vi "S2C_PCIe7841_Proc_DigitalWriteLocal.vi"(8 "Error In":errorcluster, 9 "ExeRef":refnum<vi>, 11 "Q-Ref":refnum<queue>) -> (0 "Error Out":errorcluster, 3 "Command":string)   [LabVIEW 2015]
uses:
  Typedefs/S2C_PCIe7841_Type_Conn0Write.ctl
  Typedefs/S2C_PCIe7841_Type_Conn1Write.ctl
  Typedefs/S2C_PCIe7841_Type_Conn2Write.ctl
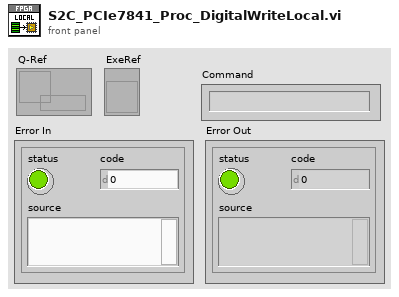
[diagram p1: front panel]
types:
  T1 = cluster{"Caller-Q":refnum<queue>, "Command":string, "Return":string, "Data":variant, "Timeout":dbl}
  T2 = typedef "S2C_PCIe7841_Type_Conn0Write.ctl" = u16
  T3 = typedef "S2C_PCIe7841_Type_Conn1Write.ctl" = u16
  T4 = typedef "S2C_PCIe7841_Type_Conn2Write.ctl" = u16
  T5 = cluster{"Connector":u16, "Conn0_Item":T2, "Conn1_Item":T3, "Conn2_Item":T4, "State":bool, "P5C1Exe":bool}
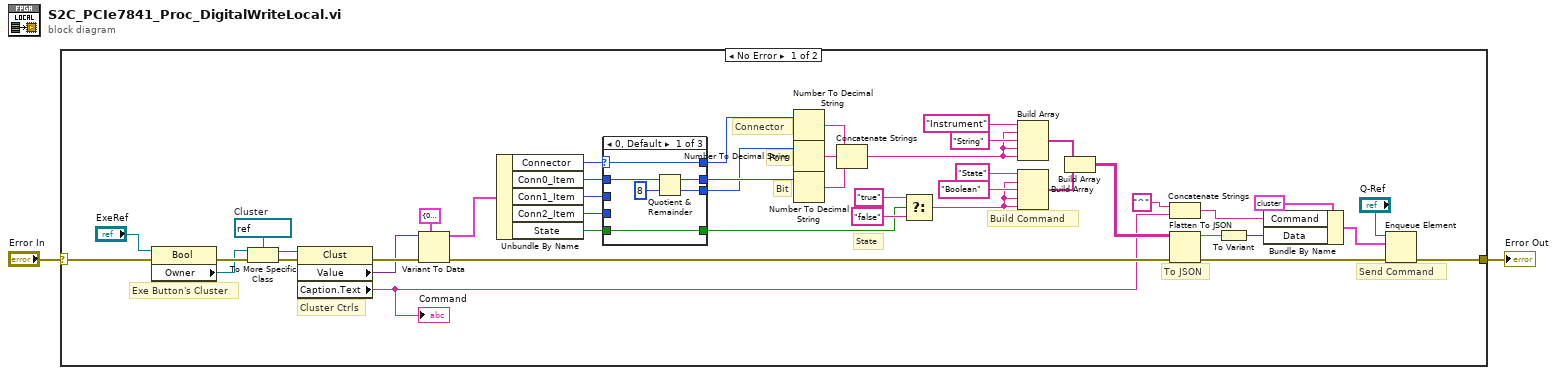
[diagram p0: block diagram]
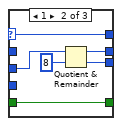
[diagram p2: hidden frame]
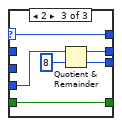
[diagram p3: hidden frame]
diagram:
  n1 = case shown="No Error" "Error In" {
    selector: "Error In" -> [w41 w66]
    tunnel: [w40 w66] -> w1
    frame No Error {
      w44 = refnum<vi> refnum  # Cluster
      # "Build Command"
      # "State"
      # "Bit"
      # "Port"
      # "Connector"
      # "Send Command"
      # "To JSON"
      # "Cluster Ctrls"
      # "Exe Button's Cluster"
      n2 = property class="Bool"(reference="ExeRef", error in=w41) -> (error out=w46:errorcluster, "Owner"=w45:refnum<vi>)  [unwired: 1 out]
      n3 = To More Specific Class(target class=w44, reference=w45, error in=w46) -> (specific class reference=w42:refnum<vi>, error out=w43:errorcluster)
      n4 = property class="Clust"(reference=w42, error in=w43) -> (error out=w39:errorcluster, "Value"=w38:variant, "Caption.Text"=w3:string)  [unwired: 1 out]
      "Command" <- w3
      n5 = Variant To Data(error in=w39, type=T5 {"Connector"=0, "Conn0_Item"=0, "Conn1_Item"=0, "Conn2_Item"=0, "State"=TRUE, "P5C1Exe"=FALSE} ("Digital Write"), Variant=w38) -> (data=w25:T5, error out=w13:errorcluster)
      n6 = Unbundle By Name(w25) -> ("Connector"=w36:u16, "Conn0_Item"=w35:T2, "Conn1_Item"=w28:T3, "Conn2_Item"=w27:T4, "State"=w26:bool)
      n7 = case shown="0, Default" w36 {
        selector: w36 -> [w52 w59 w65]
        tunnel: w35 -> [w53 _ _]
        tunnel: [w52 w59 w65] -> w34
        tunnel: [w51 w58 w64] -> w30
        tunnel: [w50 w57 w63] -> w29
        tunnel: w28 -> [_ w55 _]
        tunnel: w27 -> [_ _ w61]
        tunnel: w26 -> [w48 w54 w60]
        tunnel: [w48 w54 w60] -> w8
        frame 0, Default {
          n8 = Quotient & Remainder(x=w53, y=8) -> (x-y*floor(x/y)=w51:i32, floor(x/y)=w50:i32)
        }
        frame 1 {
          n9 = Quotient & Remainder(x=w55, y=8) -> (x-y*floor(x/y)=w58:i32, floor(x/y)=w57:i32)
        }
        frame 2 {
          n10 = Quotient & Remainder(x=w61, y=8) -> (x-y*floor(x/y)=w64:i32, floor(x/y)=w63:i32)
        }
      }
      n11 = Number To Decimal String(number=w34) -> (decimal integer string=w31:string)  [unwired: 1 in]
      n12 = Number To Decimal String(number=w29) -> (decimal integer string=w33:string)  [unwired: 1 in]
      n13 = Number To Decimal String(number=w30) -> (decimal integer string=w32:string)  [unwired: 1 in]
      n14 = Concatenate Strings(w31, w33, w32) -> (w14:string)
      n15 = Select(t="true", s=w8, f="false") -> (s? t:f=w7:string)
      n16 = Build Array("Instrument" ("element"), w14, "String" ("element"), w14, w14) -> (w6:string[])
      n17 = Build Array("State" ("element"), w7, "Boolean" ("element"), w7, w7) -> (w5:string[])
      n18 = Build Array(w6, w5) -> (w4:string[][])
      n19 = Concatenate Strings("^" ("string"), w3) -> (w21:string)
      n20 = Flatten To JSON(anything=w4, error in (no error)=w13) -> (JSON string=w23:string, 11:w24:errorcluster)  [unwired: 1 in]
      n21 = To Variant(anything=w23) -> (Variant=w19:variant)
      n22 = Bundle By Name(cluster=T1 {"Caller-Q"=refnum, "Command"="", "Return"="None", "Data"=variant, "Timeout"=10.0} ("element"), "Command"=w21, "Data"=w19) -> (w18:T1)
      n23 = Enqueue Element(queue="Q-Ref", element=w18, error in (no error)=w24) -> (error out=w40:errorcluster)  [unwired: 1 in, 2 out]
    }
    frame Error {
    }
  }
  "Error Out" <- w1
